vi "BRig_RT__Case_Exp__storeData__endExp__v5__p2__wait.vi"(0 "input_dataCurrent":u16[](array[numeric]), 1 "input_dataLick":u16[][](array[numeric]), 7 "input_True":bool=TRUE, 9 "input_dataTrial":u16[][](array[numeric]), 11 "input_dataMTrig":u16[](array[numeric])) -> (8 "output_True":bool)   [LabVIEW 2014]
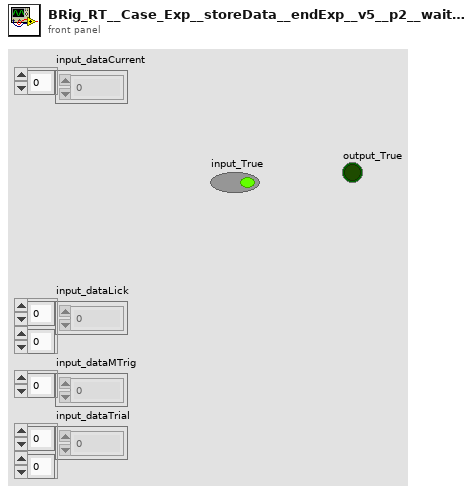
[diagram p1: front panel]
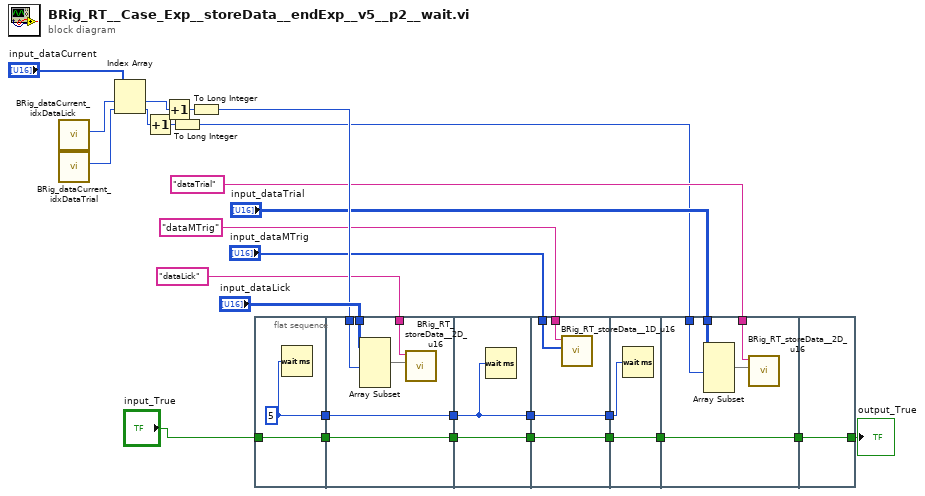
[diagram p0: block diagram]
diagram:
  n1 = call "BRig_dataCurrent_idxDataLick.vi"() -> ("output_idxDataLick"=w18:i32)  [unwired: 11 in]
  n2 = call "BRig_dataCurrent_idxDataTrial.vi"() -> ("output_idxDataTrial"=w17:i32)  [unwired: 11 in]
  n3 = Index Array(array="input_dataCurrent", index #1=w18, index #2=w17) -> (element #1=w16:u16, element #2=w13:u16)
  n4 = Increment(x=w13) -> (x+1=w14:u16)
  n5 = Increment(x=w16) -> (x+1=w15:u16)
  n6 = To Long Integer(number=w14) -> (32bit integer=w19:i32)
  n7 = To Long Integer(number=w15) -> (32bit integer=w25:i32)
  n8 = flat-sequence {
    tunnel: [w29] -> w10
    tunnel: "input_True" -> [w29]
    tunnel: [w28] -> w4
    tunnel: "input_dataLick" -> [w35]
    tunnel: w25 -> [w34]
    tunnel: "dataLick" ("input_filename") -> [w32]
    tunnel: [w31] -> w8
    tunnel: w10 -> [w31]
    tunnel: w4 -> [w30]
    tunnel: [w30] -> w3
    tunnel: w8 -> [w37]
    tunnel: [w37] -> w7
    tunnel: w3 -> [w36]
    tunnel: [w36] -> w2
    tunnel: "input_dataMTrig" -> [w41]
    tunnel: "dataMTrig" ("input_filename") -> [w40]
    tunnel: [w39] -> w6
    tunnel: w7 -> [w39]
    tunnel: w2 -> [w38]
    tunnel: [w38] -> w1
    tunnel: w6 -> [w43]
    tunnel: [w43] -> w5
    tunnel: w1 -> [w42]
    tunnel: "input_dataTrial" -> [w48]
    tunnel: "dataTrial" ("input_filename") -> [w46]
    tunnel: w19 -> [w45]
    tunnel: [w44] -> w12
    tunnel: w5 -> [w44]
    tunnel: [w49] -> w11
    tunnel: w12 -> [w49]
    frame #0 {
      w28 = u32 5 ("milliseconds to wait")
      n9 = Wait (ms)(milliseconds to wait=w28) -> ()  [unwired: 1 out]
    }
    frame #1 {
      n10 = Array Subset(array=w35, length (row)=w34) -> (w33:u16[][])  [unwired: 3 in]
      n11 = call "BRig_RT_storeData__2D_u16.vi"("Array"=w33, "input_filename"=w32) -> ()  [unwired: 10 in]
    }
    frame #2 {
      n12 = Wait (ms)(milliseconds to wait=w36) -> ()  [unwired: 1 out]
    }
    frame #3 {
      n13 = call "BRig_RT_storeData__1D_u16.vi"("Array"=w41, "input_filename"=w40) -> ()  [unwired: 10 in]
    }
    frame #4 {
      n14 = Wait (ms)(milliseconds to wait=w42) -> ()  [unwired: 1 out]
    }
    frame #5 {
      n15 = Array Subset(array=w48, length (row)=w45) -> (w47:u16[][])  [unwired: 3 in]
      n16 = call "BRig_RT_storeData__2D_u16.vi"("Array"=w47, "input_filename"=w46) -> ()  [unwired: 10 in]
    }
    frame #6 {
    }
  }
  "output_True" <- w11
